vi "SetFilter.vi"(1 "FilterSettings":T1, 2 "DeviceNumber":i32) -> (0 "success":i32)   [LabVIEW 2009]
panel:
  in  "FilterFlag":u32
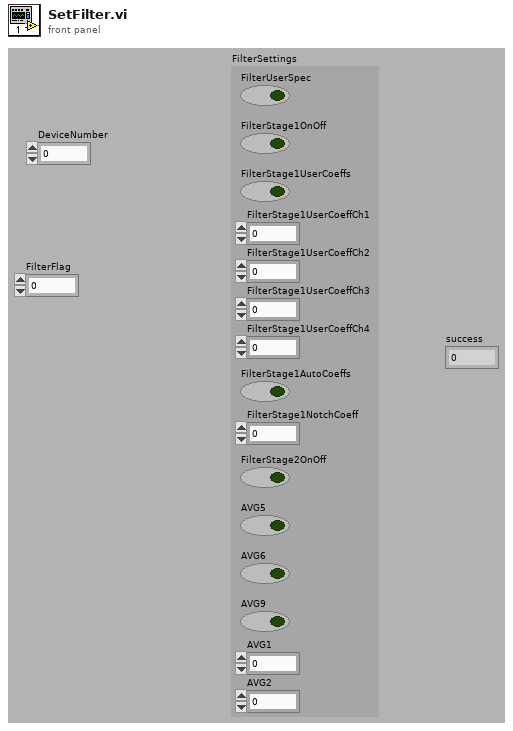
[diagram p1: front panel]
types:
  T1 = cluster{"FilterUserSpec":bool, "FilterStage1OnOff":bool, "FilterStage1UserCoeffs":bool, "FilterStage1UserCoeffCh1":dbl, "FilterStage1UserCoeffCh2":dbl, "FilterStage1UserCoeffCh3":dbl, "FilterStage1UserCoeffCh4":dbl, "FilterStage1AutoCoeffs":bool, "FilterStage1NotchCoeff":dbl, "FilterStage2OnOff":bool, "AVG5":bool, "AVG6":bool, "AVG9":bool, "AVG1":u8, "AVG2":u8}
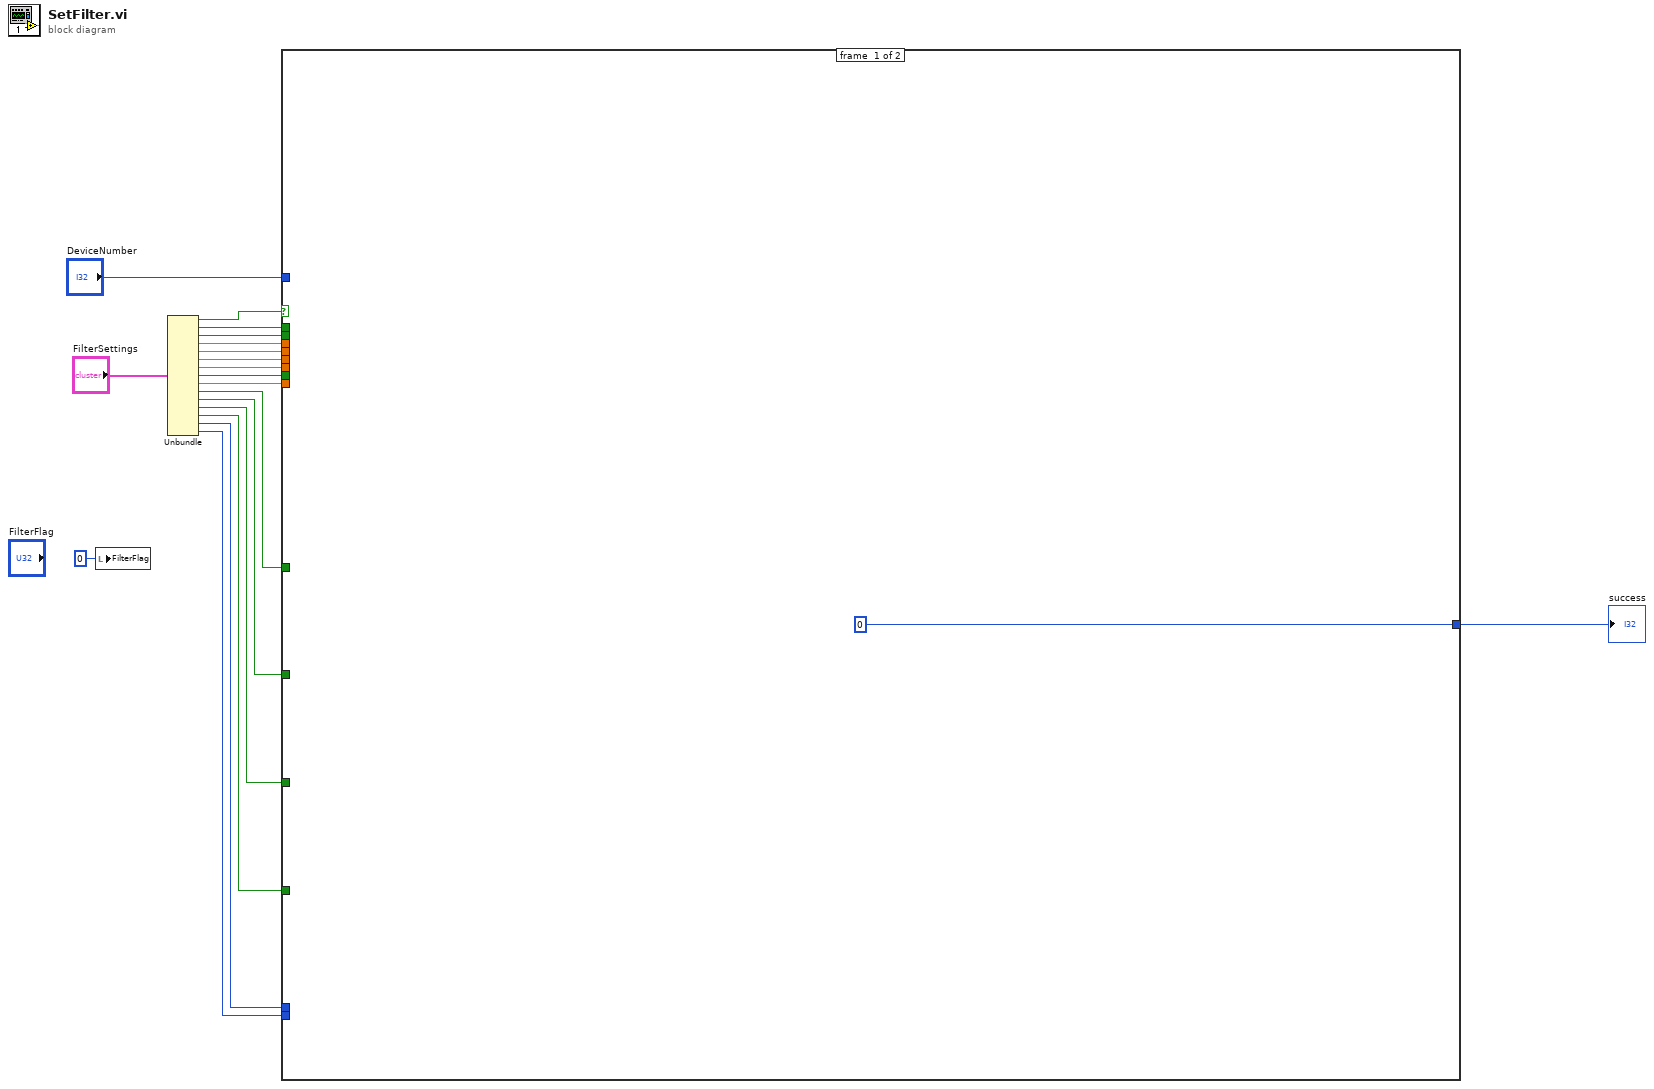
[diagram p0: block diagram]
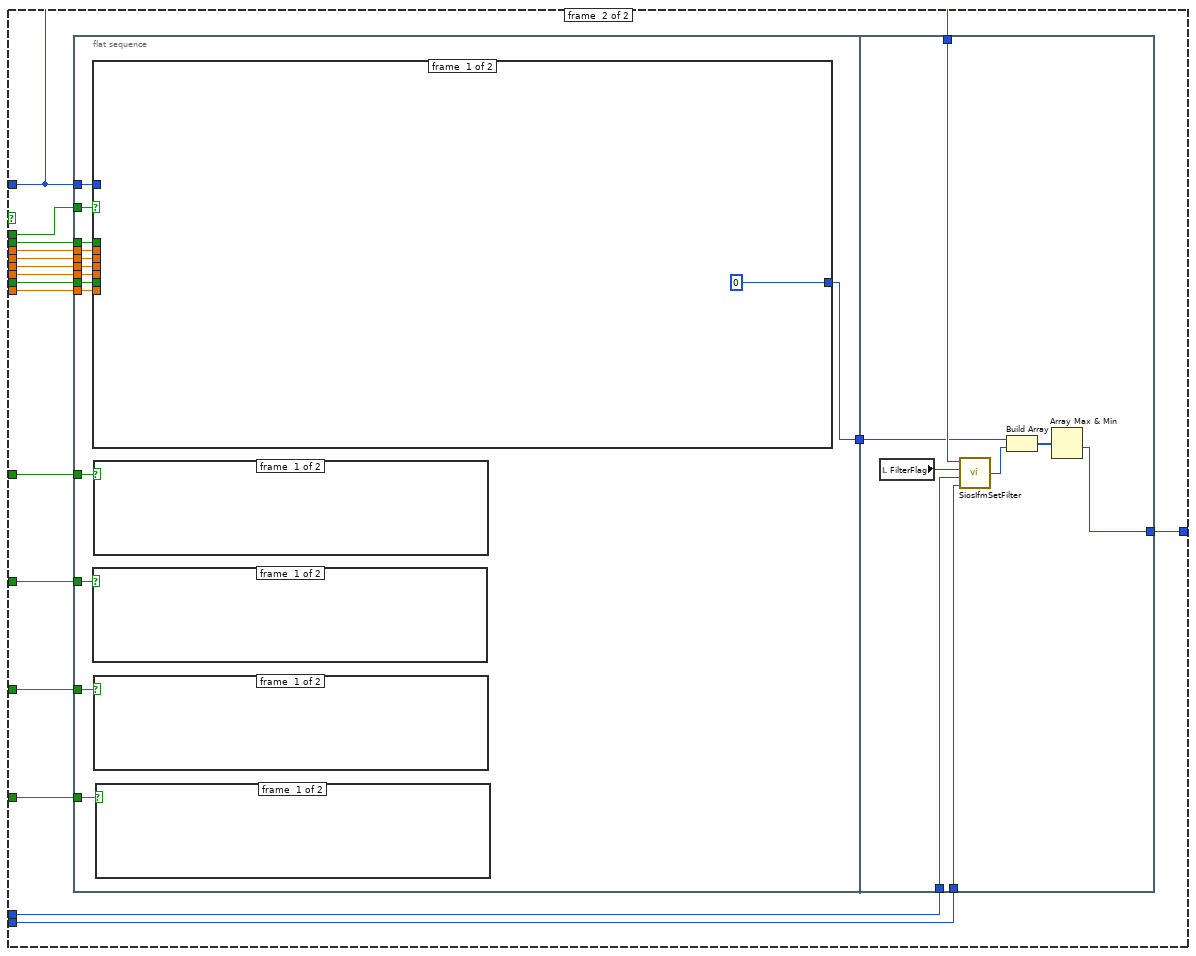
[diagram p2: hidden frame]
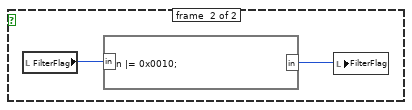
[diagram p3: hidden frame]
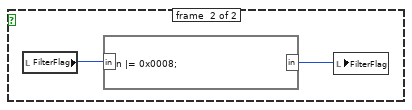
[diagram p4: hidden frame]
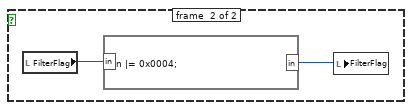
[diagram p5: hidden frame]
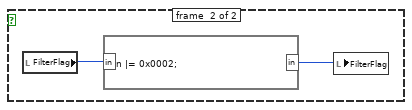
[diagram p6: hidden frame]
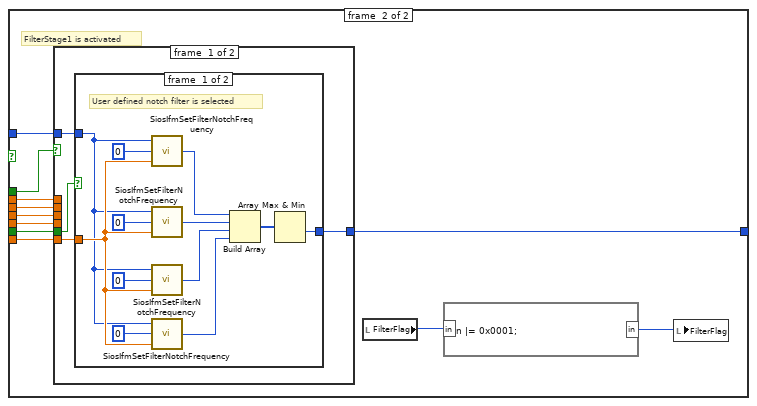
[diagram p7: hidden frame]
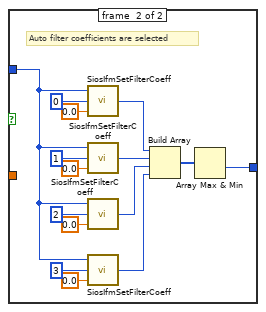
[diagram p8: hidden frame]
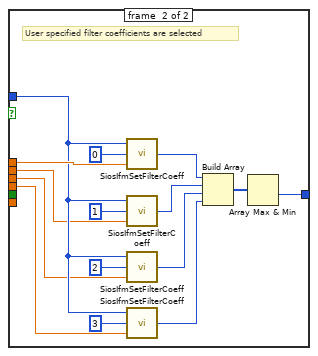
[diagram p9: hidden frame]
diagram:
  n1 = local write "FilterFlag"(u32 0 ("FilterFlag")) -> ()
  n2 = Unbundle("FilterSettings") -> ("FilterUserSpec"=w18:bool, "FilterStage1OnOff"=w16:bool, "FilterStage1UserCoeffs"=w15:bool, "FilterStage1UserCoeffCh1"=w14:dbl, "FilterStage1UserCoeffCh2"=w13:dbl, "FilterStage1UserCoeffCh3"=w12:dbl, "FilterStage1UserCoeffCh4"=w11:dbl, "FilterStage1AutoCoeffs"=w10:bool, "FilterStage1NotchCoeff"=w9:dbl, "FilterStage2OnOff"=w8:bool, "AVG5"=w7:bool, "AVG6"=w6:bool, "AVG9"=w5:bool, "AVG1"=w4:u8, "AVG2"=w3:u8)
  n3 = case shown="True" w18 {
    tunnel: [0 w21] -> w17
    tunnel: w16 -> [_ w37]
    tunnel: w15 -> [_ w36]
    tunnel: w14 -> [_ w35]
    tunnel: w13 -> [_ w34]
    tunnel: w12 -> [_ w33]
    tunnel: w11 -> [_ w32]
    tunnel: w10 -> [_ w31]
    tunnel: w9 -> [_ w30]
    tunnel: w8 -> [_ w29]
    tunnel: w7 -> [_ w28]
    tunnel: w6 -> [_ w27]
    tunnel: w5 -> [_ w26]
    tunnel: w4 -> [_ w24]
    tunnel: w3 -> [_ w23]
    tunnel: "DeviceNumber" -> [_ w25]
    frame #0 {
    }
    frame #1 {
      n4 = flat-sequence {
        tunnel: w37 -> [w51]
        tunnel: w36 -> [w50]
        tunnel: w35 -> [w49]
        tunnel: w34 -> [w48]
        tunnel: w33 -> [w47]
        tunnel: w32 -> [w46]
        tunnel: w31 -> [w45]
        tunnel: w25 -> [w44]
        tunnel: w30 -> [w43]
        tunnel: w29 -> [w42]
        tunnel: w28 -> [w41]
        tunnel: w27 -> [w40]
        tunnel: w26 -> [w39]
        tunnel: [w38] -> w22
        tunnel: w25 -> [w125]
        tunnel: w24 -> [w123]
        tunnel: w23 -> [w122]
        tunnel: w22 -> [w120]
        tunnel: [w118] -> w21
        frame #0 {
          n5 = case shown="True" w51 {
            tunnel: w50 -> [_ w71]
            tunnel: w49 -> [_ w69]
            tunnel: w48 -> [_ w67]
            tunnel: w47 -> [_ w66]
            tunnel: w46 -> [_ w65]
            tunnel: w45 -> [_ w70]
            tunnel: w44 -> [_ w68]
            tunnel: w43 -> [_ w62]
            tunnel: [0 w61] -> w38
            frame #0 {
            }
            frame #1 {
              # "FilterStage1 is activated"
              n6 = case shown="False" w71 {
                tunnel: w70 -> [w75 _]
                tunnel: w69 -> [_ w116]
                tunnel: w68 -> [w74 w115]
                tunnel: w67 -> [_ w114]
                tunnel: w66 -> [_ w113]
                tunnel: w65 -> [_ w112]
                tunnel: w62 -> [w73 _]
                tunnel: [w72 w103] -> w61
                frame #0 {
                  n7 = case shown="False" w75 {
                    tunnel: w74 -> [w79 w95]
                    tunnel: w73 -> [w80 _]
                    tunnel: [w85 w89] -> w72
                    frame #0 {
                      # "User defined notch filter is selected"
                      n8 = call "SiosIfmSetFilterNotchFrequency.vi"("FilterStage1NotchCoeff"=w80, "channel"=0, "DeviceNumber"=w79) -> ("success"=w87:i32)
                      n9 = call "SiosIfmSetFilterNotchFrequency.vi"("FilterStage1NotchCoeff"=w80, "channel"=0, "DeviceNumber"=w79) -> ("success"=w78:i32)
                      n10 = call "SiosIfmSetFilterNotchFrequency.vi"("FilterStage1NotchCoeff"=w80, "channel"=0, "DeviceNumber"=w79) -> ("success"=w77:i32)
                      n11 = call "SiosIfmSetFilterNotchFrequency.vi"("FilterStage1NotchCoeff"=w80, "channel"=0, "DeviceNumber"=w79) -> ("success"=w76:i32)
                      n12 = Build Array(w87, w78, w77, w76) -> (w86:i32[])
                      n13 = Array Max & Min(array=w86) -> (min value=w85:i32)  [unwired: 3 out]
                    }
                    frame #1 {
                      # "Auto filter coefficients are selected"
                      n14 = call "SiosIfmSetFilterCoeff.vi"("FilterStage1UserCoeffCh1"=0.0, "channel"=0, "DeviceNumber"=w95) -> ("success"=w94:i32)
                      n15 = call "SiosIfmSetFilterCoeff.vi"("FilterStage1UserCoeffCh1"=0.0, "channel"=1, "DeviceNumber"=w95) -> ("success"=w93:i32)
                      n16 = call "SiosIfmSetFilterCoeff.vi"("FilterStage1UserCoeffCh1"=0.0, "channel"=2, "DeviceNumber"=w95) -> ("success"=w91:i32)
                      n17 = call "SiosIfmSetFilterCoeff.vi"("FilterStage1UserCoeffCh1"=0.0, "channel"=3, "DeviceNumber"=w95) -> ("success"=w92:i32)
                      n18 = Build Array(w94, w93, w91, w92) -> (w90:i32[])
                      n19 = Array Max & Min(array=w90) -> (min value=w89:i32)  [unwired: 3 out]
                    }
                  }
                }
                frame #1 {
                  # "User specified filter coefficients are selected"
                  n20 = call "SiosIfmSetFilterCoeff.vi"("FilterStage1UserCoeffCh1"=w116, "channel"=0, "DeviceNumber"=w115) -> ("success"=w107:i32)
                  n21 = call "SiosIfmSetFilterCoeff.vi"("FilterStage1UserCoeffCh1"=w114, "channel"=1, "DeviceNumber"=w115) -> ("success"=w106:i32)
                  n22 = call "SiosIfmSetFilterCoeff.vi"("FilterStage1UserCoeffCh1"=w113, "channel"=2, "DeviceNumber"=w115) -> ("success"=w104:i32)
                  n23 = call "SiosIfmSetFilterCoeff.vi"("FilterStage1UserCoeffCh1"=w112, "channel"=3, "DeviceNumber"=w115) -> ("success"=w105:i32)
                  n24 = Build Array(w107, w106, w104, w105) -> (w108:i32[])
                  n25 = Array Max & Min(array=w108) -> (min value=w103:i32)  [unwired: 3 out]
                }
              }
              n26 = local read "FilterFlag"() -> (w64:u32)
              n27 = formula code="in |= 0x0001;"("in"=w64) -> ("in"=w63:u32)
              n28 = local write "FilterFlag"(w63) -> ()
            }
          }
          n29 = case shown="True" w41 {
            frame #0 {
            }
            frame #1 {
              n30 = local read "FilterFlag"() -> (w56:u32)
              n31 = formula code="in |= 0x0004;"("in"=w56) -> ("in"=w57:u32)
              n32 = local write "FilterFlag"(w57) -> ()
            }
          }
          n33 = case shown="True" w42 {
            frame #0 {
            }
            frame #1 {
              n34 = local read "FilterFlag"() -> (w58:u32)
              n35 = formula code="in |= 0x0002;"("in"=w58) -> ("in"=w59:u32)
              n36 = local write "FilterFlag"(w59) -> ()
            }
          }
          n37 = case shown="True" w40 {
            frame #0 {
            }
            frame #1 {
              n38 = local read "FilterFlag"() -> (w54:u32)
              n39 = formula code="in |= 0x0008;"("in"=w54) -> ("in"=w55:u32)
              n40 = local write "FilterFlag"(w55) -> ()
            }
          }
          n41 = case shown="True" w39 {
            frame #0 {
            }
            frame #1 {
              n42 = local read "FilterFlag"() -> (w52:u32)
              n43 = formula code="in |= 0x0010;"("in"=w52) -> ("in"=w53:u32)
              n44 = local write "FilterFlag"(w53) -> ()
            }
          }
        }
        frame #1 {
          n45 = local read "FilterFlag"() -> (w124:u32)
          n46 = call "SiosIfmSetFilter.vi"("AVG2"=w122, "AVG1"=w123, "FilterFlag"=w124, "DeviceNumber"=w125) -> ("success"=w121:i32)
          n47 = Build Array(w120, w121) -> (w119:i32[])
          n48 = Array Max & Min(array=w119) -> (min value=w118:i32)  [unwired: 3 out]
        }
      }
    }
  }
  "success" <- w17
